vi "Configure Two Tone.vi"(7 "Enable Two Tones (T:Enable)":bool=TRUE, 8 "error in (no error)":errorcluster, 9 "Frequency Spacing (10 kHz)":dbl=10000.0, 10 "Alignment (0: Left)":u16(ring) items=["Left", "Center", "Right"], 11 "VISA resource name":refnum<visa-resource-name>) -> (0 "error out":errorcluster, 3 "VISA resource name out":refnum<visa-resource-name>)   [LabVIEW 2014, in "Agilent PSG MXG Series.lvlib"]
doc: "Configures the state, alignment type and frequency spacing of the two-tone waveform generator.\n\n<B>Notes:</B>\n(1) This VI is valid only in E8267C, E8267D, N5162A, N5182A, N5172B, N5182B.\n\n(2) For E8267C, this VI is valid only when the instrument installs <B>Option 002</B> (Internal baseband generator) or <B>Option 602</B> (Digital bus baseband generator).\n\n(3) For E8267D, this VI is valid only when the instrument installs <B>Option 601</B> or <B>Option 602</B> (Internal baseband generator).\n\n(4) For N5162A and N5182A, this VI is valid only when the instrument installs <B>Option 651</B> or <B>Option 652</B> or <B>Option 654</B> (Internal baseband generator), and <B>Option 430</B> (Multitone and two-tone)."
uses:
  Agilent PSG MXG Series.lvlib
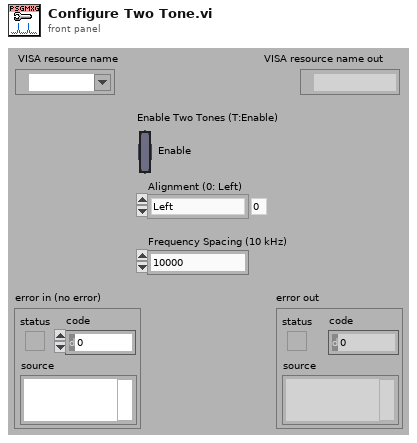
[diagram p1: front panel]
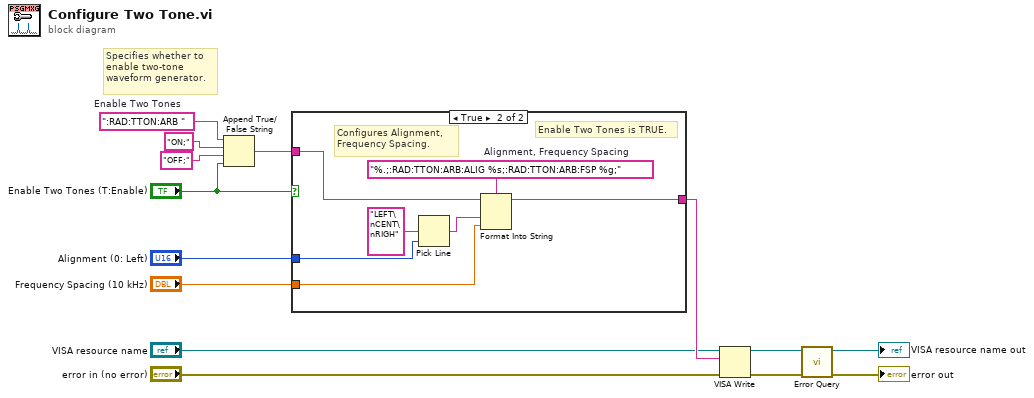
[diagram p0: block diagram]
diagram:
  w14 = ":RAD:TTON:ARB "  # Enable Two Tones
  # "Specifies whether to\nenable two-tone\nwaveform generator."
  n1 = Append True/False String(1:"Enable Two Tones (T:Enable)", 2:"OFF;" ("false string"), 3:"ON;" ("true string"), 4:w14) -> (0:w10:string)
  n2 = case shown="True" "Enable Two Tones (T:Enable)" {
    tunnel: w10 -> [w15 w22]
    tunnel: "Alignment (0: Left)" -> [_ w19]
    tunnel: "Frequency Spacing (10 kHz)" -> [_ w17]
    tunnel: [w15 w16] -> w7
    frame False {
      # "Enable Two Tones is FALSE."
    }
    frame True {
      w21 = "%.;:RAD:TTON:ARB:ALIG %s;:RAD:TTON:ARB:FSP %g;"  # Alignment, Frequency Spacing
      # "Configures Alignment,\nFrequency Spacing."
      # "Enable Two Tones is TRUE."
      n3 = Pick Line(multi-line string="LEFT\nCENT\nRIGH", line index=w19) -> (output string=w18:string)  [unwired: 1 out]
      n4 = Format Into String(format string=w21, initial string=w22, w18, w17) -> (resulting string=w16:string)  [unwired: 1 in, 1 out]
    }
  }
  n5 = VISA Write(VISA resource name="VISA resource name", write buffer=w7, error in (no error)="error in (no error)") -> (VISA resource name out=w6:refnum<visa-resource-name>, error out=w5:errorcluster)  [unwired: 1 out]
  n6 = call "Error Query.vi"("error in (no error)"=w5, "VISA resource name"=w6) -> ("error out"=→"error out":errorcluster, "VISA resource name out"=→"VISA resource name out":refnum<visa-resource-name>)  [unwired: 8 out]
